vi "Uart timeout.vi"(7 "timeout ms (2000)":i32=2000, 8 "error in":errorcluster, 10 "Timeout (*0.1s)":u8, 11 "RedPitaya connection in":refnum<k5>) -> (0 "error out":errorcluster, 3 "RedPitaya connection out":refnum<k5>)   [LabVIEW 2021]
uses:
  Variance measurement/Red_Pitaya/RedPitaya.lvlib
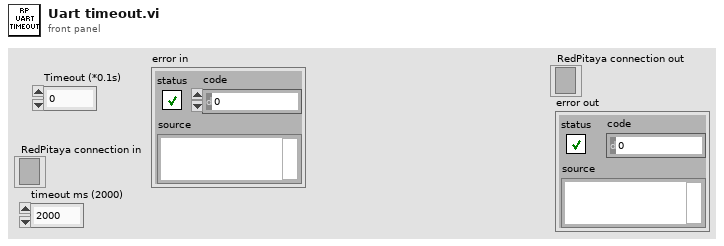
[diagram p1: front panel]
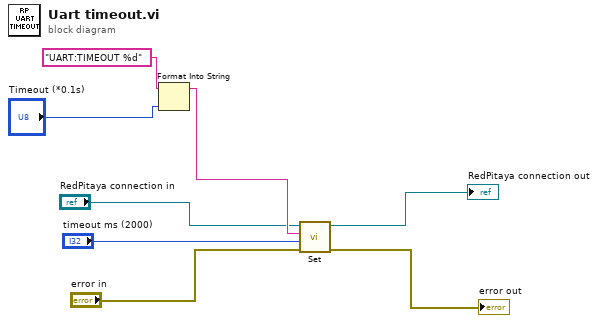
[diagram p0: block diagram]
diagram:
  n1 = Format Into String(format string="UART:TIMEOUT %d", "Timeout (*0.1s)") -> (resulting string=w7:string)  [unwired: 2 in, 1 out]
  n2 = call "Set.vi"("error in"="error in", "timeout ms (2000)"="timeout ms (2000)", "SCPI Message"=w7, "RedPitaya connection in"="RedPitaya connection in") -> ("error out"=→"error out":errorcluster, "RedPitaya connection out"=→"RedPitaya connection out":refnum<k5>)  [unwired: 5 in, 1 out]
